vi "Adjust Power.vi"(11 "D-pad input":dbl) -> ()   [LabVIEW 2014]
uses:
  Events.vi
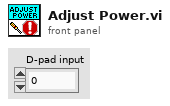
[diagram p1: front panel]
types:
  T1 = cluster{"Reloading?":bool, "Throw":bool, "Ready?":bool, "Truss throw":bool, "Power is high?":bool, "Automatic relaod?":bool, "Manuall servo":bool}
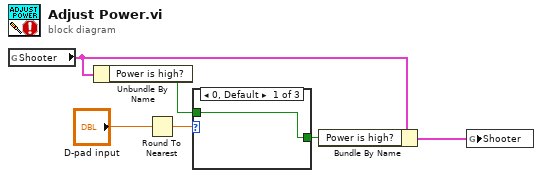
[diagram p0: block diagram]
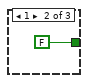
[diagram p2: hidden frame]
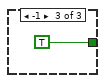
[diagram p3: hidden frame]
diagram:
  n1 = global read "Events.vi" "Shooter"() -> (w4:T1)
  n2 = Unbundle By Name(w4) -> ("Power is high?"=w3:bool)
  n3 = Round To Nearest(number="D-pad input") -> (nearest integer value=w1:dbl)
  n4 = case shown="0, Default" w1 {
    tunnel: [w7 FALSE TRUE] -> w5
    tunnel: w3 -> [w7 _ _]
    frame 0, Default {
    }
    frame 1 {
    }
    frame -1 {
    }
  }
  n5 = Bundle By Name(cluster=w4, "Power is high?"=w5) -> (w6:T1)
  n6 = global write "Events.vi" "Shooter"(w6) -> ()
